vi "Write.vi"(4 "Append? [F]":bool, 6 "File Type":T1, 8 "error in (no error)":errorcluster, 9 "Notes":string, 10 "Data (Dictionary)":T2[](array[typedef]), 11 "path":path) -> (0 "error out":errorcluster, 3 "path out":path)   [LabVIEW 2016, in "Data.lvclass"]
uses:
  Data.lvclass
  Typedefs/Dictionary--cluster.ctl
  Typedefs/Type--enum.ctl
  Data.lvclass/Data.ctl
  Data.DAT/Data.DAT.lvclass
  C:/user/patrick/git/LV-to-ITX/src/Data/Data.lvclass
  Data.ITX/Data.ITX.lvclass
  Data.HDF5/Data.HDF5.lvclass
  Data.TDMS/Data.TDMS.lvclass
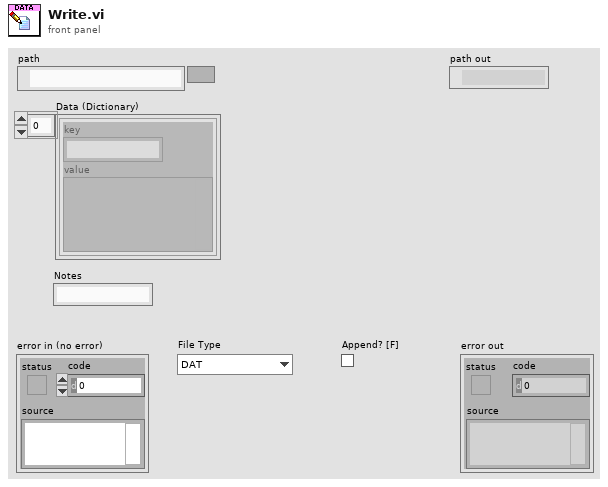
[diagram p1: front panel]
types:
  T1 = typedef "Data.lvclass/Type--enum.ctl" = enum16{"DAT", "ITX", "HDF5", "TDMS", "VI"}
  T2 = typedef "Data.lvclass/Dictionary--cluster.ctl" = cluster{"key":string, "value":variant}
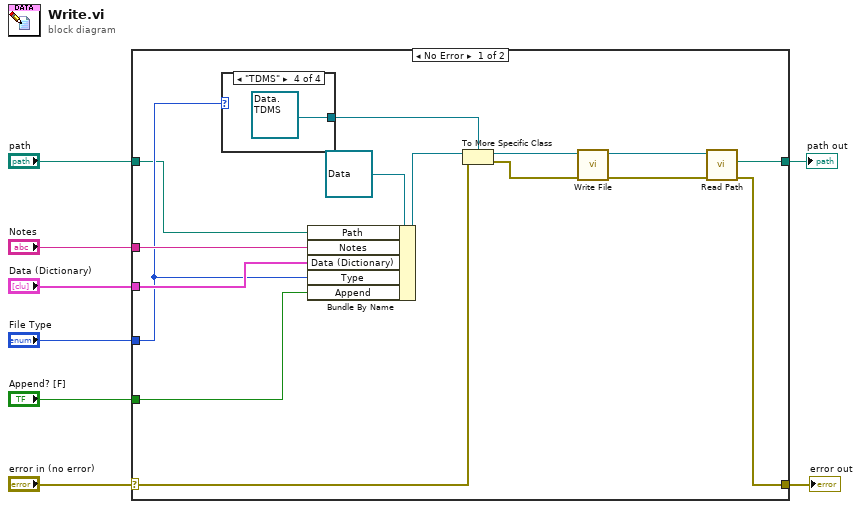
[diagram p0: block diagram]
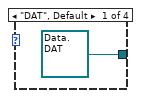
[diagram p2: hidden frame]
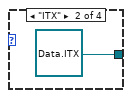
[diagram p3: hidden frame]
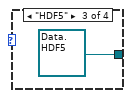
[diagram p4: hidden frame]
diagram:
  n1 = case shown="No Error" "error in (no error)" {
    selector: "error in (no error)" -> [w18 w29]
    tunnel: [w22 w29] -> w7
    tunnel: "path" -> [w10 w28]
    tunnel: "Data (Dictionary)" -> [w16 _]
    tunnel: "Notes" -> [w17 _]
    tunnel: "File Type" -> [w15 _]
    tunnel: "Append? [F]" -> [w9 _]
    tunnel: [w23 w28] -> w2
    frame No Error {
      n2 = case shown="\"TDMS\"" w15 {
        tunnel: [refnum<class "Data.DAT.lvclass"> refnum ("Data.DAT.lvclass") refnum<class "Data.ITX.lvclass"> refnum ("Data.ITX.lvclass") refnum<class "Data.HDF5.lvclass"> refnum ("Data.HDF5.lvclass") refnum<class "Data.TDMS.lvclass"> refnum ("Data.TDMS.lvclass")] -> w21
        frame "DAT", Default {
        }
        frame "ITX" {
        }
        frame "HDF5" {
        }
        frame "TDMS" {
        }
      }
      n3 = Bundle By Name(cluster=refnum<class "Data.lvclass"> refnum ("target class"), "Path"=w10, "Notes"=w17, "Data (Dictionary)"=w16, "Type"=w15, "Append"=w9) -> (w19:refnum<class "Data.lvclass">)
      n4 = To More Specific Class(target class=w21, reference=w19, error in=w18) -> (specific class reference=w14:refnum<class "Data.lvclass">, error out=w13:errorcluster)
      n5 = call-dynamic "Write File.vi"("error in (no error)"=w13, "Data in"=w14) -> ("error out"=w12:errorcluster, "Data out"=w11:refnum<class "Data.lvclass">)  [unwired: 8 in]
      n6 = call "Read Path.vi"("error in (no error)"=w12, "Data Save"=w11) -> ("error out"=w22:errorcluster, "Path"=w23:path)  [unwired: 7 in, 1 out]
    }
    frame Error {
    }
  }
  "error out" <- w7
  "path out" <- w2
